vi "Run.vi"(8 "error in (no error)":errorcluster, 11 "socket SUB in":refnum<class "socket SUB.lvclass">) -> (0 "error out":errorcluster, 3 "socket SUB out":refnum<class "socket SUB.lvclass">)   [LabVIEW 2018, in "socket SUB.lvclass"]
uses:
  socket SUB.lvclass
  C:/Users/Denis/Desktop/communication-manager/communication-manager/Socket/Socket.lvclass
  State Machine/CM_State Machine.lvclass/CM_State Machine.ctl
  Socket/Socket.lvclass
  State Machine/CM_State Machine.lvclass
  RxTx/CM_RxTx.lvclass
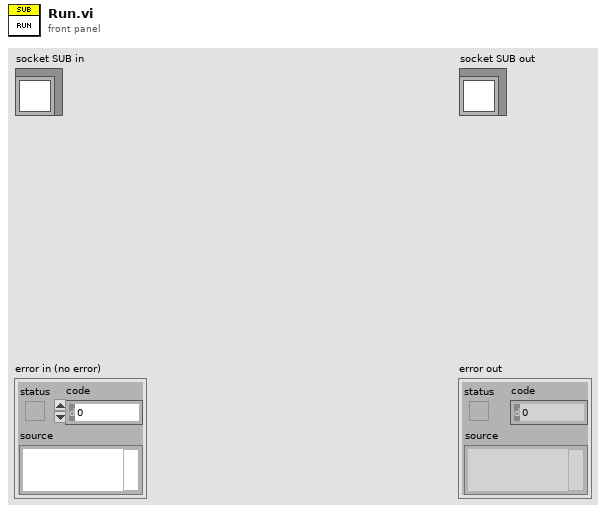
[diagram p1: front panel]
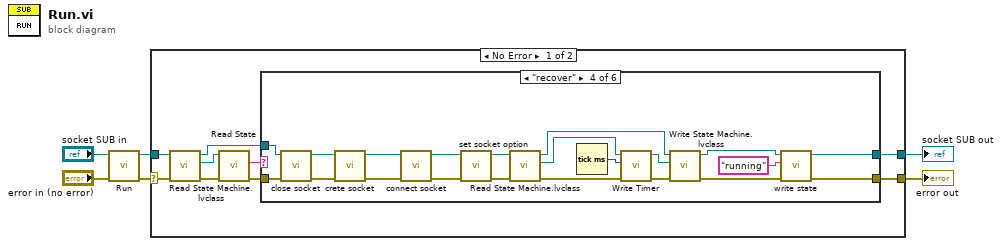
[diagram p0: block diagram]
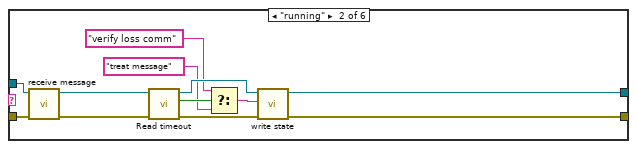
[diagram p3: hidden frame]
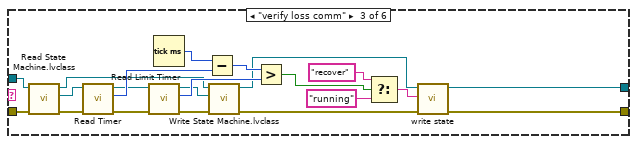
[diagram p4: hidden frame]
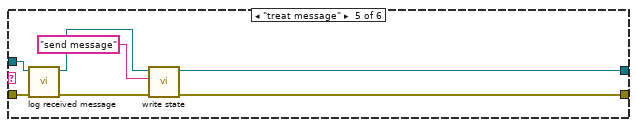
[diagram p5: hidden frame]
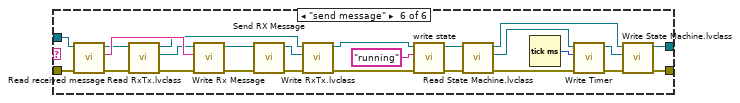
[diagram p6: hidden frame]
diagram:
  n1 = call-parent "Run.vi"("error in (no error)"="error in (no error)", "Socket in"="socket SUB in") -> ("error out"=w3:errorcluster, "Socket out"=w4:refnum<class "socket SUB.lvclass">)  [unwired: 8 in]
  n2 = case shown="No Error" w3 {
    selector: w3 -> [w9 w104]
    tunnel: w4 -> [w10 w105]
    tunnel: [w13 w105] -> w2
    tunnel: [w14 w104] -> w1
    frame No Error {
      n3 = call-dynamic "Read State Machine.lvclass.vi"("error in (no error)"=w9, "Socket in"=w10) -> ("error out"=w8:errorcluster, "State Machine.lvclass"=w11:refnum<class "CM_State Machine.lvclass">, "Socket out"=w7:refnum<class "socket SUB.lvclass">)  [unwired: 7 in]
      n4 = call-dynamic "Read State.vi"("error in (no error)"=w8, "State Machine in"=w11) -> ("error out"=w12:errorcluster, "State"=w15:string)  [unwired: 7 in, 1 out]
      n5 = case shown="\"recover\"" w15 {
        tunnel: [w16 w26 w49 w70 w73 w82] -> w13
        tunnel: [w17 w27 w50 w71 w72 w83] -> w14
        tunnel: w12 -> [w17 w28 w44 w67 w76 w89]
        tunnel: w7 -> [w16 w29 w45 w68 w75 w90]
        frame Default {
        }
        frame "running" {
          n6 = call-dynamic "receive message.vi"("error in (no error)"=w28, "Socket in"=w29) -> ("error out"=w25:errorcluster, "Socket out"=w24:refnum<class "socket SUB.lvclass">)  [unwired: 8 in]
          n7 = call-dynamic "Read timeout.vi"("error in (no error)"=w25, "Socket in"=w24) -> ("error out"=w22:errorcluster, "timeout"=w21:bool, "Socket out"=w23:refnum<class "socket SUB.lvclass">)  [unwired: 7 in]
          n8 = Select(t="verify loss comm", s=w21, f="treat message" ("t")) -> (s? t:f=w20:string)
          n9 = call "write state.vi"("error in (no error)"=w22, "State"=w20, "Socket in"=w23) -> ("error out"=w27:errorcluster, "Socket out"=w26:refnum<class "socket SUB.lvclass">)  [unwired: 7 in]
        }
        frame "verify loss comm" {
          n10 = call-dynamic "Read State Machine.lvclass.vi"("error in (no error)"=w44, "Socket in"=w45) -> ("error out"=w43:errorcluster, "State Machine.lvclass"=w42:refnum<class "CM_State Machine.lvclass">, "Socket out"=w30:refnum<class "socket SUB.lvclass">)  [unwired: 7 in]
          n11 = call "Read Timer.vi"("error in (no error)"=w43, "State Machine in"=w42) -> ("error out"=w37:errorcluster, "Timer"=w40:u32, "State Machine out"=w36:refnum<class "CM_State Machine.lvclass">)  [unwired: 7 in]
          n12 = call "Read Limit Timer.vi"("error in (no error)"=w37, "State Machine in"=w36) -> ("error out"=w32:errorcluster, "Limit Timer"=w39:u32, "State Machine out"=w31:refnum<class "CM_State Machine.lvclass">)  [unwired: 7 in]
          n13 = Tick Count (ms)() -> (millisecond timer value=w41:u32)
          n14 = Subtract(x=w41, y=w40) -> (x-y=w38:u32)
          n15 = call-dynamic "Write State Machine.lvclass.vi"("error in (no error)"=w32, "State Machine.lvclass"=w31, "Socket in"=w30) -> ("error out"=w33:errorcluster, "Socket out"=w34:refnum<class "socket SUB.lvclass">)  [unwired: 7 in]
          n16 = Greater?(x=w38, y=w39) -> (0:w35:bool)
          n17 = Select(t="recover", s=w35, f="running" ("t")) -> (s? t:f=w48:string)
          n18 = call "write state.vi"("error in (no error)"=w33, "State"=w48, "Socket in"=w34) -> ("error out"=w50:errorcluster, "Socket out"=w49:refnum<class "socket SUB.lvclass">)  [unwired: 7 in]
        }
        frame "recover" {
          n19 = call "close socket.vi"("error in (no error)"=w67, "Socket in"=w68) -> ("error out"=w63:errorcluster, "Socket out"=w66:refnum<class "socket SUB.lvclass">)  [unwired: 8 in]
          n20 = call "crete socket.vi"("error in (no error)"=w63, "Socket in"=w66) -> ("error out"=w64:errorcluster, "Socket out"=w65:refnum<class "socket SUB.lvclass">)  [unwired: 8 in]
          n21 = call "connect socket.vi"("error in (no error)"=w64, "Socket in"=w65) -> ("error out"=w61:errorcluster, "Socket out"=w62:refnum<class "socket SUB.lvclass">)  [unwired: 8 in]
          n22 = call "set socket option.vi"("error in (no error)"=w61, "Socket2 in"=w62) -> ("error out"=w53:errorcluster, "Socket2 out"=w54:refnum<class "socket SUB.lvclass">)  [unwired: 8 in]
          n23 = call-dynamic "Read State Machine.lvclass.vi"("error in (no error)"=w53, "Socket in"=w54) -> ("error out"=w57:errorcluster, "State Machine.lvclass"=w60:refnum<class "CM_State Machine.lvclass">, "Socket out"=w58:refnum<class "socket SUB.lvclass">)  [unwired: 7 in]
          n24 = Tick Count (ms)() -> (millisecond timer value=w55:u32)
          n25 = call "Write Timer.vi"("error in (no error)"=w57, "Timer"=w55, "State Machine in"=w60) -> ("error out"=w56:errorcluster, "State Machine out"=w59:refnum<class "CM_State Machine.lvclass">)  [unwired: 7 in]
          n26 = call-dynamic "Write State Machine.lvclass.vi"("error in (no error)"=w56, "State Machine.lvclass"=w59, "Socket in"=w58) -> ("error out"=w52:errorcluster, "Socket out"=w51:refnum<class "socket SUB.lvclass">)  [unwired: 7 in]
          n27 = call "write state.vi"("error in (no error)"=w52, "State"="running" ("t"), "Socket in"=w51) -> ("error out"=w71:errorcluster, "Socket out"=w70:refnum<class "socket SUB.lvclass">)  [unwired: 7 in]
        }
        frame "treat message" {
          n28 = call "log received message.vi"("error in (no error)"=w76, "Socket in"=w75) -> ("error out"=w74:errorcluster, "Socket out"=w78:refnum<class "socket SUB.lvclass">)  [unwired: 8 in]
          n29 = call "write state.vi"("error in (no error)"=w74, "State"="send message", "Socket in"=w78) -> ("error out"=w72:errorcluster, "Socket out"=w73:refnum<class "socket SUB.lvclass">)  [unwired: 7 in]
        }
        frame "send message" {
          n30 = call-dynamic "Read received message.vi"("error in (no error)"=w89, "Socket in"=w90) -> ("error out"=w95:errorcluster, "received message"=w102:string, "Socket out"=w99:refnum<class "socket SUB.lvclass">)  [unwired: 7 in]
          n31 = call-dynamic "Read RxTx.lvclass.vi"("error in (no error)"=w95, "Socket in"=w99) -> ("error out"=w94:errorcluster, "RxTx.lvclass"=w100:refnum<class "CM_RxTx.lvclass">, "Socket out"=w97:refnum<class "socket SUB.lvclass">)  [unwired: 7 in]
          n32 = call "Write Rx Message.vi"("error in (no error)"=w94, "Rx Message"=w102, "RxTx in"=w100) -> ("error out"=w101:errorcluster, "RxTx out"=w103:refnum<class "CM_RxTx.lvclass">)  [unwired: 7 in]
          n33 = call "Send RX Message.vi"("error in (no error)"=w101, "RxTx in"=w103) -> ("error out"=w96:errorcluster, "RxTx out"=w98:refnum<class "CM_RxTx.lvclass">)  [unwired: 8 in]
          n34 = call-dynamic "Write RxTx.lvclass.vi"("error in (no error)"=w96, "RxTx.lvclass"=w98, "Socket in"=w97) -> ("error out"=w93:errorcluster, "Socket out"=w92:refnum<class "socket SUB.lvclass">)  [unwired: 7 in]
          n35 = call "write state.vi"("error in (no error)"=w93, "State"="running", "Socket in"=w92) -> ("error out"=w81:errorcluster, "Socket out"=w80:refnum<class "socket SUB.lvclass">)  [unwired: 7 in]
          n36 = call-dynamic "Read State Machine.lvclass.vi"("error in (no error)"=w81, "Socket in"=w80) -> ("error out"=w85:errorcluster, "State Machine.lvclass"=w88:refnum<class "CM_State Machine.lvclass">, "Socket out"=w86:refnum<class "socket SUB.lvclass">)  [unwired: 7 in]
          n37 = Tick Count (ms)() -> (millisecond timer value=w79:u32)
          n38 = call "Write Timer.vi"("error in (no error)"=w85, "Timer"=w79, "State Machine in"=w88) -> ("error out"=w84:errorcluster, "State Machine out"=w87:refnum<class "CM_State Machine.lvclass">)  [unwired: 7 in]
          n39 = call-dynamic "Write State Machine.lvclass.vi"("error in (no error)"=w84, "State Machine.lvclass"=w87, "Socket in"=w86) -> ("error out"=w83:errorcluster, "Socket out"=w82:refnum<class "socket SUB.lvclass">)  [unwired: 7 in]
        }
      }
    }
    frame Error {
    }
  }
  "error out" <- w1
  "socket SUB out" <- w2
